vi "Calculate Color Index Array.vi"(8 "error in (no error)":errorcluster, 10 "3D Quiver Datatype in":refnum<class "3D Quiver Datatype.lvclass">, 11 "Plot Representation In":T1) -> (0 "error out":errorcluster, 2 "3D Quiver Datatype out":refnum<class "3D Quiver Datatype.lvclass">, 3 "Plot Representation Out":T1)   [LabVIEW 2020, in "3D Quiver Datatype.lvclass"]
uses:
  <vilib>/Math Plots/3D Math Plots/3D Quiver/3D Quiver Datatype/3D Quiver Datatype.lvclass
  <vilib>/Math Plots/3D Math Plots/3D Plot/3D Plot/Typedef/Plot Representation.ctl
  <vilib>/Math Plots/3D Math Plots/3D Plot/3D Plot/Typedef/Range Clusters.ctl
  <vilib>/Math Plots/3D Math Plots/3D Plot/3D Plot/Typedef/Mesh Data.ctl
  <vilib>/Math Plots/3D Math Plots/3D Quiver/3D Quiver Datatype/3D Quiver Datatype.lvclass/3D Quiver Datatype.ctl
  <vilib>/Math Plots/3D Math Plots/3D Plot/3D Plot Datatype/3D Plot Datatype.lvclass
  <vilib>/Math Plots/3D Math Plots/3D Plot/3D Plot/3D Plot.lvclass
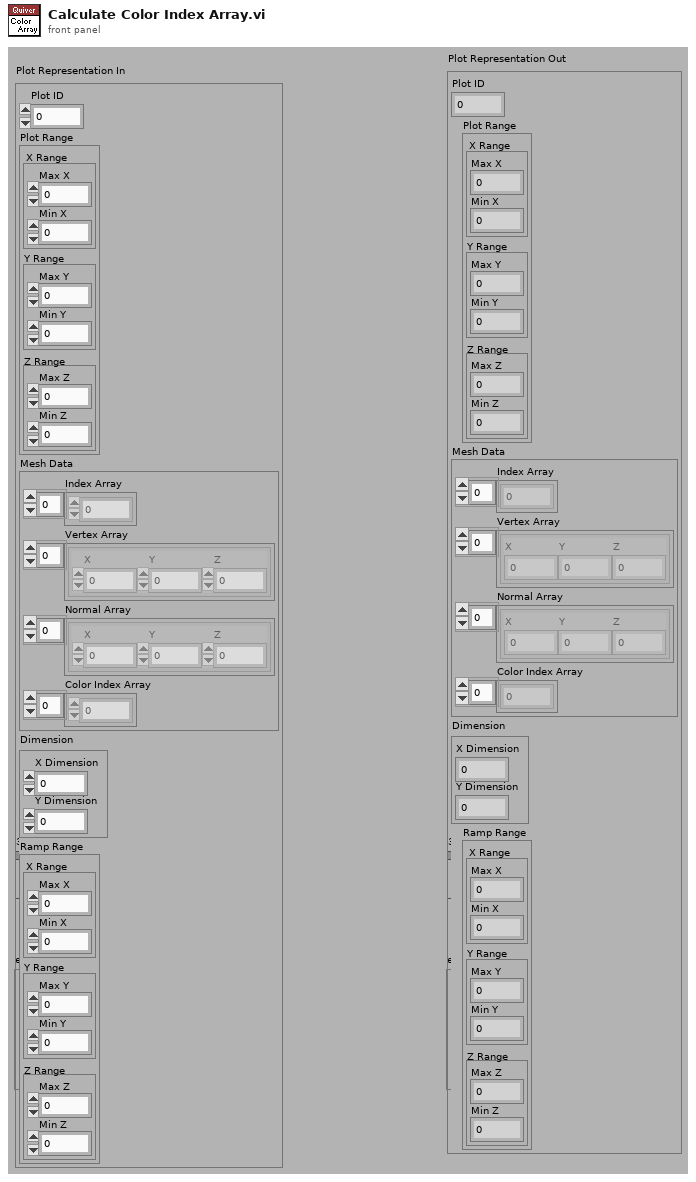
[diagram p1: front panel]
types:
  T1 = typedef "3D Plot.lvclass/Plot Representation.ctl" = cluster{"Plot ID":i32, "Plot Range":T2, "Mesh Data":T3, "Dimension":cluster{"X Dimension":i32, "Y Dimension":i32}, "Ramp Range":T2}
  T2 = typedef "3D Plot.lvclass/Range Clusters.ctl" = cluster{"X Range":cluster{"Max X":sgl, "Min X":sgl}, "Y Range":cluster{"Max Y":sgl, "Min Y":sgl}, "Z Range":cluster{"Max Z":sgl, "Min Z":sgl}}
  T3 = typedef "3D Plot.lvclass/Mesh Data.ctl" = cluster{"Index Array":u32[], "Vertex Array":cluster{"X":sgl, "Y":sgl, "Z":sgl}[], "Normal Array":cluster{"X":sgl, "Y":sgl, "Z":sgl}[], "Color Index Array":i32[]}
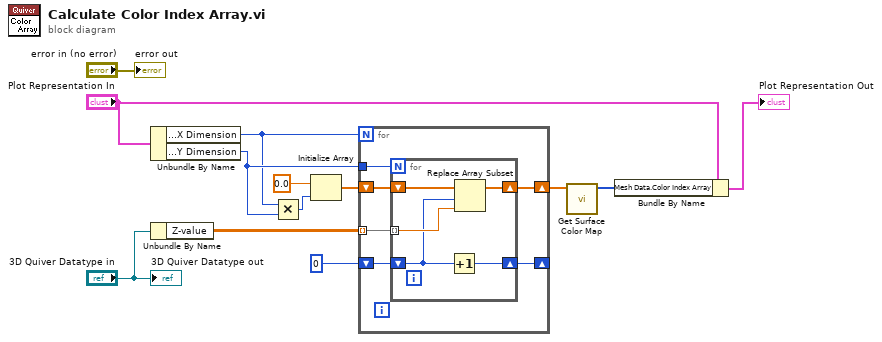
[diagram p0: block diagram]
diagram:
  n1 = Unbundle By Name("Plot Representation In") -> ("Dimension.X Dimension"=w4:i32, "Dimension.Y Dimension"=w5:i32)
  n2 = Unbundle By Name("3D Quiver Datatype in") -> ("Z-value"=w9:sgl[][])
  n3 = Multiply(x=w4, y=w5) -> (x*y=w6:i32)
  n4 = Initialize Array(sgl 0.0 ("element"), w6) -> (w8:sgl[])
  n5 = for {
    N: w4 -> [_]
    tunnel: w5 -> [w19]
    shift-right: [w14] -> w3
    shift-left: w8 -> [w18]
    tunnel: w9 -> [w17] mode=indexing
    shift-right: [w16] -> _
    shift-left: 0 -> [w15]
    n6 = for {
      N: w19 -> [_]
      shift-right: [w23] -> w14
      shift-left: w18 -> [w24]
      tunnel: w17 -> [w22] mode=indexing
      shift-right: [w21] -> w16
      shift-left: w15 -> [w20]
      n7 = Increment(x=w20) -> (x+1=w21:i32)
      n8 = Replace Array Subset(array=w24, new element=w22, index=w20) -> (w23:sgl[])
    }
  }
  n9 = call <vilib>:"Get Surface Color Map.vi"("Amplifiy"=w3) -> ("Color Index Array"=w11:i32[])  [unwired: 1 in, 9 out]
  n10 = Bundle By Name(cluster="Plot Representation In", "Mesh Data.Color Index Array"=w11) -> (→"Plot Representation Out":T1)
  "error out" <- "error in (no error)"
  "3D Quiver Datatype out" <- "3D Quiver Datatype in"
